vi "Generated Descriptors.vi"() -> (3 "Descriptor Strings":string[](array[string]))   [LabVIEW 2023, in "Generated_server.lvlib"]
uses:
  Generated_server.lvlib
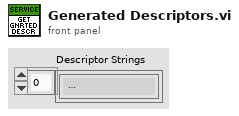
[diagram p1: front panel]
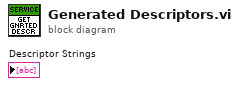
[diagram p0: block diagram]
diagram:
